vi "1L22_Rm_Uref.vi"(9 "Uref":dbl=5.0, 10 "Rc":dbl, 11 "Um":dbl) -> (3 "Rm":dbl)   [LabVIEW 2010, in "lv_01.lvlib"]
uses:
  lv_01.lvlib
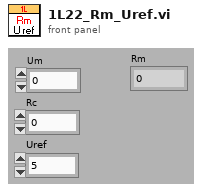
[diagram p1: front panel]
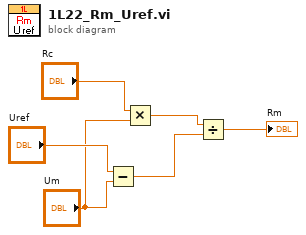
[diagram p0: block diagram]
diagram:
  n1 = Subtract(x="Uref", y="Um") -> (x-y=w1:dbl)
  n2 = Multiply(x="Rc", y="Um") -> (x*y=w2:dbl)
  n3 = Divide(x=w2, y=w1) -> (x/y=→"Rm":dbl)
